vi "Test.vi"() -> ()   [LabVIEW 2023]
uses:
  Tree/Tree.lvclass
  1ab23d85-62a6-4864-8003-68581c5663eb.vi
  ac8319fc-5c84-47ba-a3f9-734e81557296.vi
panel:
  in  "확인 버튼":bool
  in  "CSV Path":path
  in  "Tree 입력":refnum<class "Tree.lvclass">
  in  "트리":string(tree)
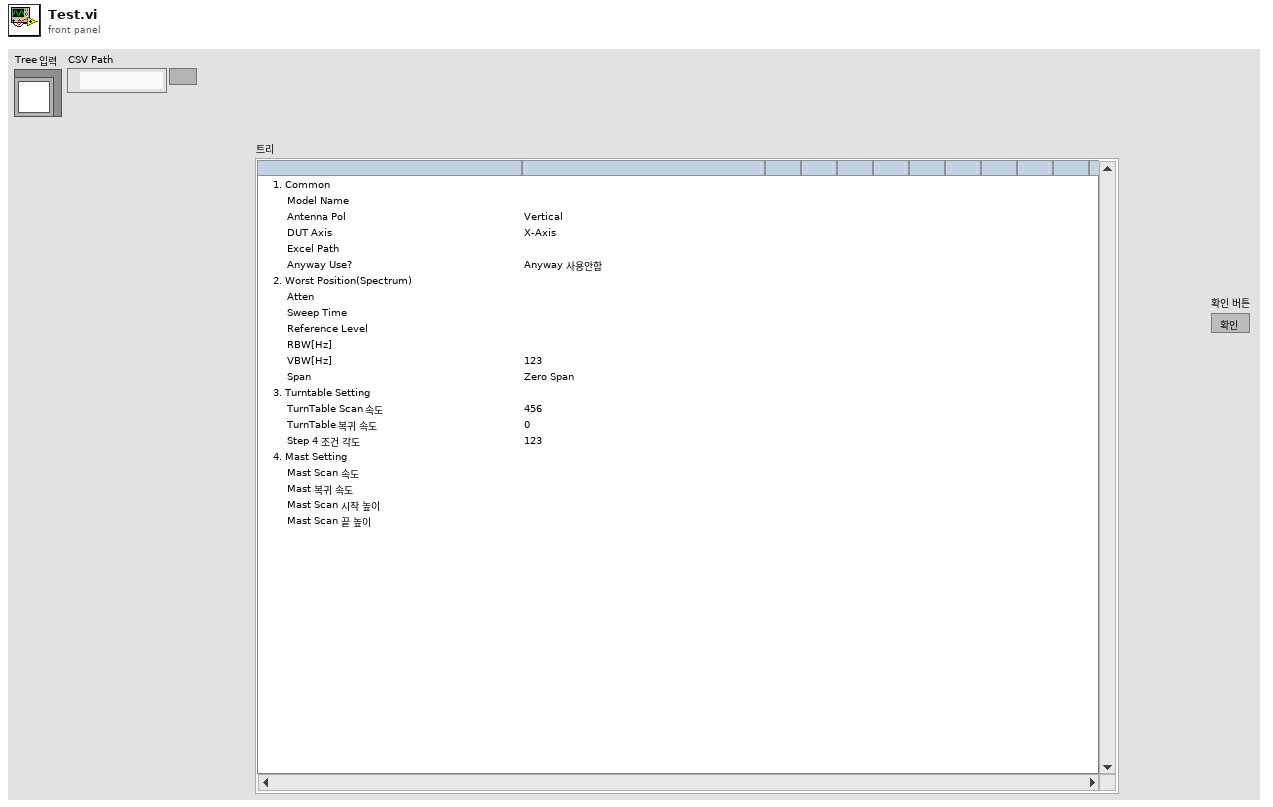
[diagram p1: front panel]
types:
  T1 = typedef "eventvkey.ctl" = enum16{"ASCII", "Enter", "Return", "Shift", "Ctrl", "Alt", "Cmd", "Opt", "Caps", "NumLock", "Clear", "Break", "Up", "Down", "Left", "Right", "Insert", "Delete", "Home", "End", "PageUp", "PageDown", "Escape", "Help", "Pause", "ScrollLock", "F1", "F2", "F3", "F4", "F5", "F6", "F7", "F8", "F9", "F10", "F11", "F12", "F13", "F14", "F15", "F16", "F17", "F18", "F19", "F20", "F21", "F22", "F23", "F24", "Play", "VolumeUp", "VolumeDown", "Mute", "Two Byte Char"}
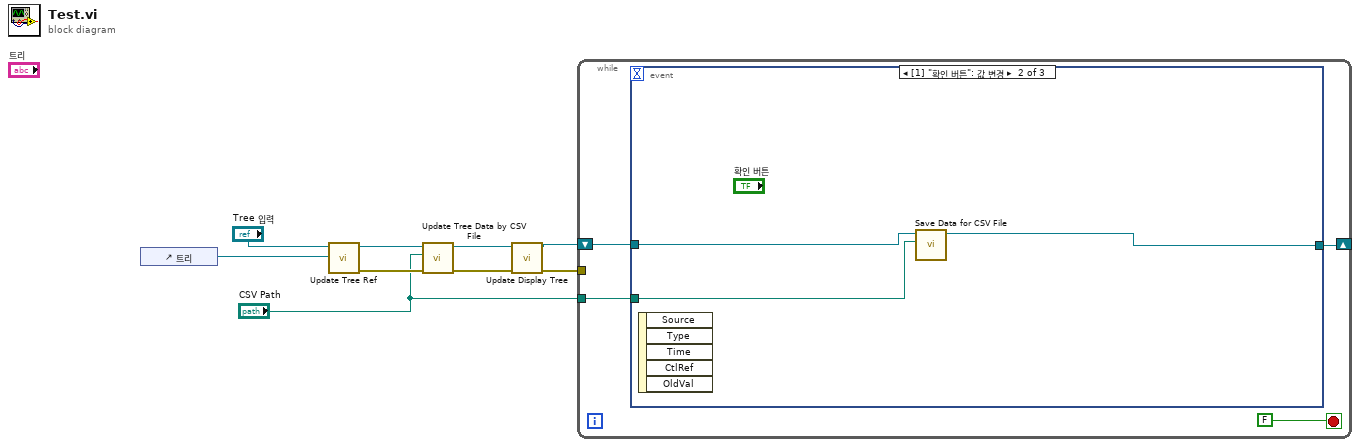
[diagram p0: block diagram]
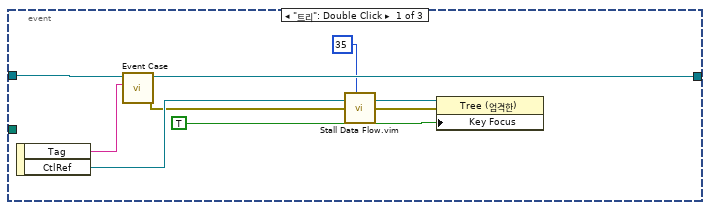
[diagram p2: hidden frame]
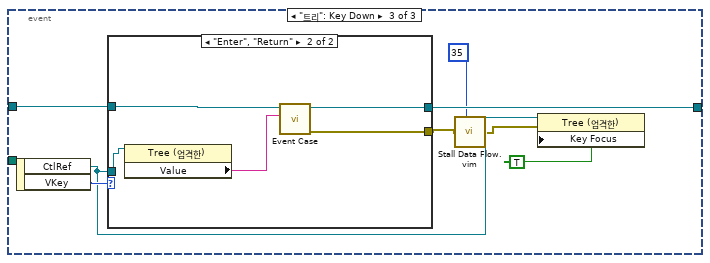
[diagram p3: hidden frame]
diagram:
  n1 = control-ref of="트리"() -> (w9:refnum<vi>)
  n2 = call "Update Tree Ref.vi"("Tree Ref"=w9, "Tree 입력"="Tree 입력") -> ("error out"=w4:errorcluster, "Tree 출력"=w7:refnum<class "Tree.lvclass">)  [unwired: 8 in]
  n3 = call "Update Tree Data by CSV File.vi"("error in (no error)"=w4, "CSV Path"="CSV Path", "Tree 입력"=w7) -> ("error out"=w5:errorcluster, "Tree 출력"=w6:refnum<class "Tree.lvclass">)  [unwired: 7 in]
  n4 = call "Update Display Tree.vi"("error in (no error)"=w5, "Tree 입력"=w6) -> ("error out"=w2:errorcluster, "Tree 출력"=w3:refnum<class "Tree.lvclass">)  [unwired: 8 in]
  n5 = while {
    tunnel: w2 -> [_]
    shift-right: [w11] -> _
    shift-left: w3 -> [w12]
    tunnel: "CSV Path" -> [w10]
    stop <- FALSE stop-if-true
    n6 = event shown="[1] \"확인 버튼\": 값 변경" {
      selector: _ -> [_ _ _]
      dyn-events: _ -> [_ _ _]
      timeout: _ -> [_ _ _]
      tunnel: w12 -> [w21 w24 w31]
      tunnel: [w17 w23 w29] -> w11
      tunnel: w10 -> [_ w22 _]
      event "트리": Double Click {
        n7 = event-data() -> ("Tag"=w20:string, "CtlRef"=w18:refnum<vi>)  [unwired: 1 in]
        n8 = call "Event Case.vi"("Event>tag"=w20, "Tree 입력"=w21) -> ("error out"=w16:errorcluster, "Tree 출력"=w17:refnum<class "Tree.lvclass">)  [unwired: 8 in]
        n9 = call "Stall Data Flow.vim"("value in"=w16, "milliseconds to wait"=u32 35) -> ("value out"=w15:errorcluster)  [unwired: 1 out]
        n10 = property class="Tree (엄격한)"(reference=w18, error in=w15, "Key Focus"=TRUE ("키 포커스")) -> ()  [unwired: 2 out]
      }
      event "확인 버튼": Value Change {
        n11 = event-data() -> ()  [unwired: 1 in, 5 out]
        n12 = call "Save Data for CSV File.vi"("경로"=w22, "Tree 입력"=w24) -> ("Tree 출력"=w23:refnum<class "Tree.lvclass">)  [unwired: 8 in, 1 out]
      }
      event "트리": Key Down {
        n13 = event-data() -> ("CtlRef"=w28:refnum<vi>, "VKey"=w32:T1)  [unwired: 1 in]
        n14 = case shown="\"Enter\", \"Return\"" w32 {
          tunnel: w31 -> [w33 w38]
          tunnel: [_ w36] -> w27
          tunnel: [w33 w35] -> w29
          tunnel: w28 -> [_ w34]
          frame "ASCII", Default {
          }
          frame "Enter", "Return" {
            n15 = property class="Tree (엄격한)"(reference=w34) -> ("Value"=w37:string)  [unwired: 1 in, 2 out]
            n16 = call "Event Case.vi"("Event>tag"=w37, "Tree 입력"=w38) -> ("error out"=w36:errorcluster, "Tree 출력"=w35:refnum<class "Tree.lvclass">)  [unwired: 8 in]
          }
        }
        n17 = call "Stall Data Flow.vim"("value in"=w27, "milliseconds to wait"=u32 35) -> ("value out"=w26:errorcluster)  [unwired: 1 out]
        n18 = property class="Tree (엄격한)"(reference=w28, error in=w26, "Key Focus"=TRUE ("키 포커스")) -> ()  [unwired: 2 out]
      }
    }
  }
